vi "Dmux.vi"(2 "in":bool, 4 "sel":bool) -> (6 "a":bool, 10 "b":bool)   [LabVIEW 2014]
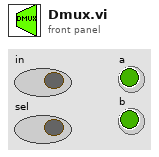
[diagram p1: front panel]
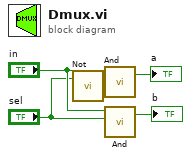
[diagram p0: block diagram]
diagram:
  n1 = call "Not.vi"("in"="sel") -> ("out"=w5:bool)  [unwired: 2 in]
  n2 = call "And.vi"("b"=w5, "a"="in") -> ("out"=→"a":bool)  [unwired: 3 in]
  n3 = call "And.vi"("b"="sel", "a"="in") -> ("out"=→"b":bool)  [unwired: 3 in]
